vi "GrabImageUDP.vi"(5 "Image in":T1, 9 "connection ID":refnum<k16>, 11 "error in":errorcluster, 12 "timeout ms (25000)":i32=200) -> (4 "Image Out":T1, 14 "error out":errorcluster, 15 "status":bool)   [LabVIEW 2013]
doc: "This vi acquires several images when it receives an external trigger signal, and extracts the one containing the beam shot. It has to be specified which type of cameras you are using, the usb ones or the RS170 ones."
uses:
  <vilib>/vision/Image Controls.llb/IMAQ Image.ctl
panel:
  out "image data string":string
  out "error timeout cleared":errorcluster
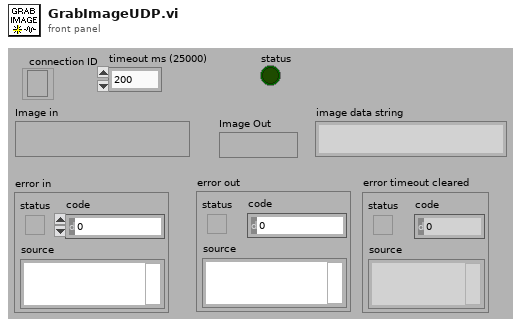
[diagram p1: front panel]
types:
  T1 = typedef "IMAQ Image.ctl" = refnum<image>
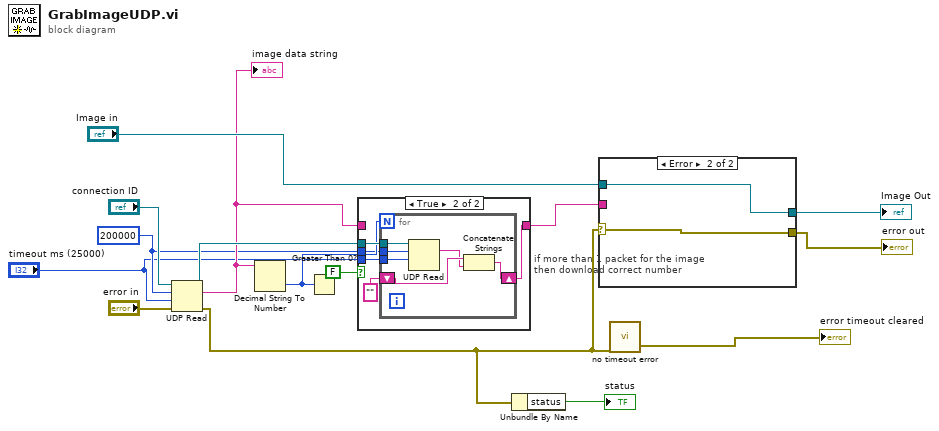
[diagram p0: block diagram]
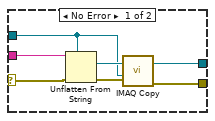
[diagram p3: hidden frame]
diagram:
  w6 = 200000 ("max size (548)")
  n1 = UDP Read(connection ID="connection ID", max size (548)=w6, timeout ms (25000)="timeout ms (25000)", 8:"error in") -> (data out=w8:string, error out=w2:errorcluster, 3:w10:refnum<k16>)  [unwired: 2 out]
  "image data string" <- w8
  n2 = Decimal String To Number(string=w8) -> (number=w9:i32)  [unwired: 2 in, 1 out]
  n3 = Greater Than 0?(x=w9) -> ()  [unwired: 1 out]
  n4 = case "if more than 1 packet for the image\nthen download correct number" shown="True" FALSE {
    tunnel: w10 -> [_ w22]
    tunnel: w9 -> [_ w21]
    tunnel: w8 -> [w16 _]
    tunnel: [w16 w18] -> w7
    tunnel: w6 -> [_ w20]
    tunnel: "timeout ms (25000)" -> [_ w19]
    frame False {
    }
    frame True {
      n5 = for {
        N: w21 -> [_]
        tunnel: w22 -> [w28]
        tunnel: w20 -> [w27]
        tunnel: w19 -> [w26]
        shift-right: [w25] -> w18
        shift-left: "" ("data out") -> [w24]
        n6 = UDP Read(connection ID=w28, max size (548)=w27, timeout ms (25000)=w26) -> (data out=w23:string)  [unwired: 1 in, 4 out]
        n7 = Concatenate Strings(w24, w23) -> (w25:string)
      }
    }
  }
  n8 = Unbundle By Name(w2) -> ("status"=→"status":bool)
  n9 = case shown="Error" w2 {
    selector: w2 -> [w31 w36]
    tunnel: w7 -> [w35 _]
    tunnel: "Image in" -> [w33 w37]
    tunnel: [w32 w37] -> w14
    tunnel: [w29 w36] -> w4
    frame No Error {
      n10 = Unflatten From String(type=w33, binary string=w35, error in (no error)=w31) -> (value=w34:T1, error out=w30:errorcluster)  [unwired: 3 out]
      n11 = call "IMAQ Copy"("error in (no error)"=w30, "Image Dst"=w33, "Image Src"=w34) -> ("error out"=w29:errorcluster, "Image Dst Out"=w32:T1)  [unwired: 3 in]
    }
    frame Error {
    }
  }
  "Image Out" <- w14
  "error out" <- w4
  n12 = call "no timeout error.vi"("error in (no error)"=w2) -> ("error out"=→"error timeout cleared":errorcluster)  [unwired: 1 out]
